vi "SR05 Example.vi"() -> ()   [LabVIEW 2012, in "LIFA Ultrasonic Distance.lvlib"]
uses:
  LIFA Ultrasonic Distance.lvlib
  <vilib>/LabVIEW Interface for Arduino/LabVIEW Interface for Arduino.lvlib
  <vilib>/LabVIEW Interface for Arduino/Type Defs/Board Type.ctl
  Get Distance/SRF05 Get Distance.vi
panel:
  in  "Mode":u16(ring) items=["Mode 1"=1, "Mode 2"=2]
  in  "stop":bool
  out "Distance History (cm)":dbl(graph)
  # "1.  Upload the provided LIFA firmware.\n\n2.  If using a board other than the Arduino UNO, change the parameters for Init.vi on the block diagram.\n\n3.  Then, select the mode that you have the SR05 wired for.\n\n4.  Run the VI.\n\nNote:  If using the SR04, use Mode 1."
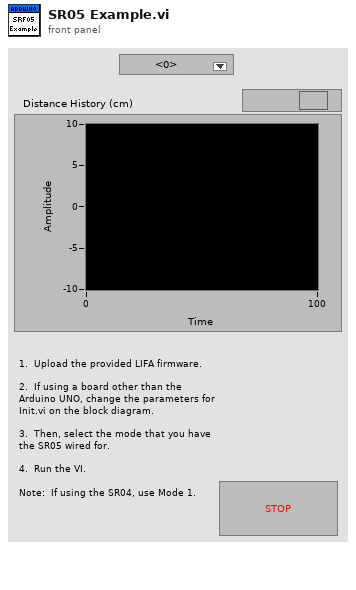
[diagram p1: front panel]
types:
  T1 = typedef "LabVIEW Interface for Arduino.lvlib/Board Type.ctl" = enum16{"Uno", "Dimuelanove w/Atmega 328", "Mega 2560"}
  T2 = typedef "LabVIEW Interface for Arduino.lvlib/Arduino Resource.ctl" = cluster{"VISA resource":refnum<visa-resource-name>, "Board Type":T1, "Connection Type":enum8{"USB / Serial"}, "Bytes Per Packet (15)":u8}
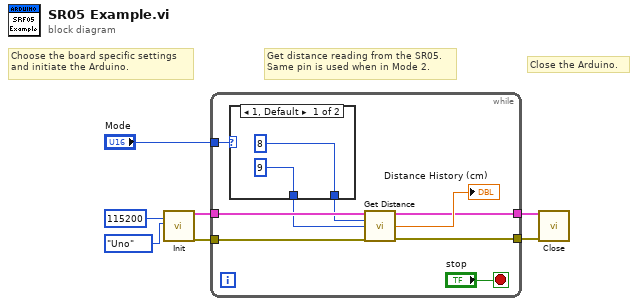
[diagram p0: block diagram]
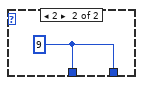
[diagram p2: hidden frame]
diagram:
  # "Close the Arduino."
  # "Get distance reading from the SR05.\nSame pin is used when in Mode 2."
  # "Choose the board specific settings\nand initiate the Arduino."
  n1 = call <vilib>:"Init.vi"("Baud Rate (115200)"=u32 115200, "Board Type (Uno)"=Board_Type."Uno") -> ("Arduino Resource"=w7:T2, "error out"=w6:errorcluster)  [unwired: 16 in]
  n2 = while {
    tunnel: w7 -> [w15]
    tunnel: w6 -> [w14]
    tunnel: [w13] -> w4
    tunnel: [w11] -> w5
    tunnel: "Mode" -> [w10]
    stop <- "stop" stop-if-true
    n3 = case shown="1, Default" w10 {
      tunnel: [u8 9 w19] -> w8
      tunnel: [u8 8 w19] -> w9
      frame 1, Default {
      }
      frame 2 {
        w19 = u8 9
      }
    }
    n4 = call-poly "Get Distance.vi"("Arduino Resource"=w15, "Trigger Pin"=w9, "Signal Pin"=w8, "error in (no error)"=w14) -> ("Arduino Resource"=w11:T2, "Distance (cm)"=→"Distance History (cm)":dbl, "error out"=w13:errorcluster)  [unwired: 9 in]
  }
  n5 = call <vilib>:"Close.vi"("Arduino Resource"=w5, "error in"=w4) -> ()  [unwired: 13 in, 1 out]
